vi "resonant volt per meter.vi"() -> (3 "volt/meter interpolated":dbl)   [LabVIEW 2012]
doc: "SciScan 1.2 160622"
uses:
  GFG/GFGnumericGet.vi
  GFG/GFGfpRefGet.vi
  GFG/GFG library.lvlib
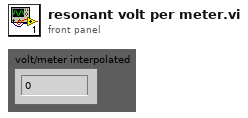
[diagram p1: front panel]
types:
  T1 = cluster{"WaveformChartRef":refnum<vi>, "DigitalRef":refnum<vi>, "ArrayRef":refnum<vi>, "TabControlRef":refnum<vi>, "EnumRef":refnum<vi>, "RingRef":refnum<vi>, "BooleanRef":refnum<vi>, "KnobRef":refnum<vi>, "SlideRef":refnum<vi>, "PathRef":refnum<vi>, "StringRef":refnum<vi>, "ComboBox":refnum<vi>, "WaveformGraphRef":refnum<vi>}
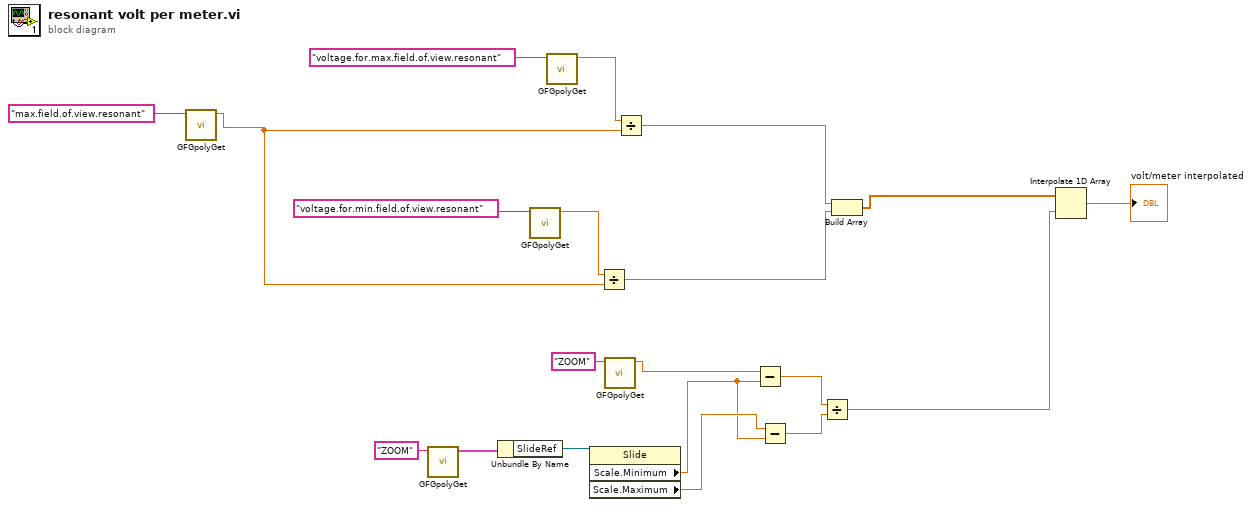
[diagram p0: block diagram]
diagram:
  n1 = call-poly "GFGpolyGet.vi"("Variable Name in"="max.field.of.view.resonant") -> ("Numeric"=w9:dbl)  [unwired: 8 in, 2 out]
  n2 = call-poly "GFGpolyGet.vi"("Variable Name in"="ZOOM") -> ("output cluster"=w12:T1)  [unwired: 9 in, 1 out]
  n3 = Unbundle By Name(w12) -> ("SlideRef"=w11:refnum<vi>)
  n4 = call-poly "GFGpolyGet.vi"("Variable Name in"="voltage.for.min.field.of.view.resonant") -> ("Numeric"=w16:dbl)  [unwired: 8 in, 2 out]
  n5 = call-poly "GFGpolyGet.vi"("Variable Name in"="voltage.for.max.field.of.view.resonant") -> ("Numeric"=w20:dbl)  [unwired: 8 in, 2 out]
  n6 = property class="Slide"(reference=w11) -> ("Scale.Minimum"=w2:dbl, "Scale.Maximum"=w3:dbl)  [unwired: 1 in, 2 out]
  n7 = Divide(x=w16, y=w9) -> (x/y=w14:dbl)
  n8 = call-poly "GFGpolyGet.vi"("Variable Name in"="ZOOM") -> ("Numeric"=w7:dbl)  [unwired: 8 in, 2 out]
  n9 = Divide(x=w20, y=w9) -> (x/y=w15:dbl)
  n10 = Subtract(x=w7, y=w2) -> (x-y=w6:dbl)
  n11 = Subtract(x=w3, y=w2) -> (x-y=w1:dbl)
  n12 = Divide(x=w6, y=w1) -> (x/y=w5:dbl)
  n13 = Build Array(w15, w14) -> (w8:dbl[])
  n14 = Interpolate 1D Array(1:w5, 2:w8) -> (0:→"volt/meter interpolated":dbl)
